vi "Read Multiple.vi"(8 "error in (no error)":errorcluster, 10 "Names":string[](array[string]), 11 "TwinCAT ADS in":refnum<class "TwinCAT ADS.lvclass">) -> (0 "error out":errorcluster, 1 "Values":variant[](array[variant]), 3 "TwinCAT ADS out":refnum<class "TwinCAT ADS.lvclass">)   [LabVIEW 2018, in "TwinCAT ADS.lvclass"]
uses:
  TwinCAT ADS.lvclass
  TwinCAT.Ads
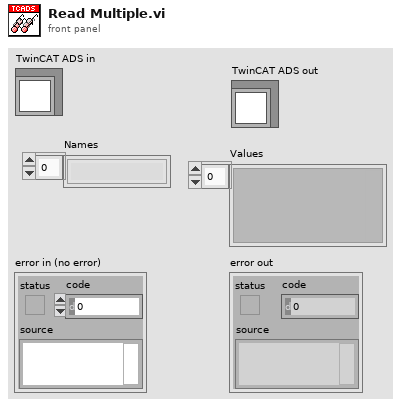
[diagram p1: front panel]
types:
  T1 = typedef "TwinCAT ADS.lvclass/Symbol Information.ctl" = cluster{"Name":string, "Short Name":string, "Size":i32, "Type Category":i32, "Type Name":string, "Type ID":i32, "Index Group":i64, "Index Offset":i64, "Child Count":i32, "Has Rpc Methods?":bool, "Comment":string}
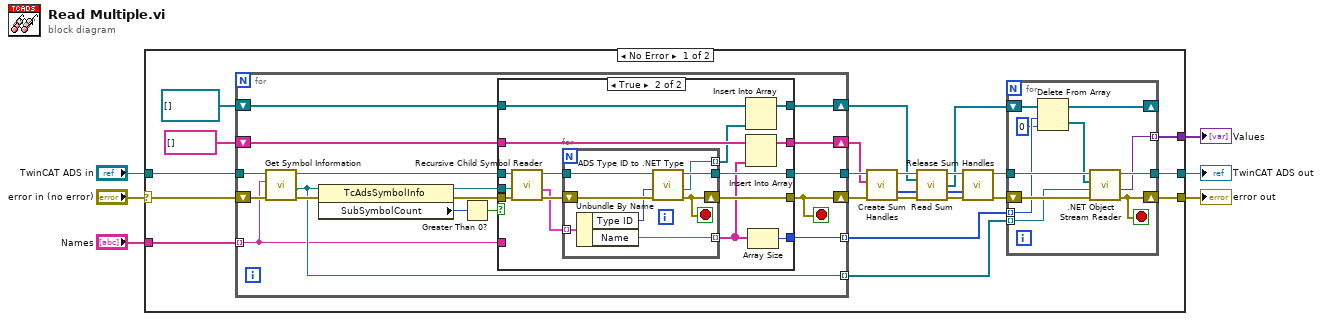
[diagram p0: block diagram]
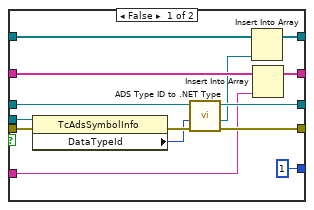
[diagram p2: hidden frame]
diagram:
  n1 = case shown="No Error" "error in (no error)" {
    selector: "error in (no error)" -> [w7 w96]
    tunnel: [w14 w96] -> w5
    tunnel: [w13 w95] -> w3
    tunnel: "TwinCAT ADS in" -> [w8 w95]
    tunnel: "Names" -> [w24 _]
    tunnel: [w12 _] -> w1
    frame No Error {
      n2 = for {
        tunnel: w24 -> [w41] mode=indexing
        shift-right: [w53] -> w26
        shift-left: string[] [] -> [w54]
        shift-right: [w52] -> w28
        shift-left: w7 -> [w46]
        tunnel: w8 -> [w45]
        tunnel: [w51] -> w27
        shift-right: [w48] -> w10
        shift-left: refnum<k24>[] [] (".NET Type Stream") -> [w50]
        tunnel: [w43] -> w11 mode=indexing
        tunnel: [w47] -> w15 mode=indexing
        stop <- w52 stop-if-true
        n3 = call-dynamic "Get Symbol Information.vi"("error in (no error)"=w46, "Name"=w41, "TwinCAT ADS in"=w45) -> ("error out"=w44:errorcluster, "Symbol Info"=w43:refnum<k24>, "TwinCAT ADS out"=w42:refnum<class "TwinCAT ADS.lvclass">)  [unwired: 6 in]
        n4 = property class="TcAdsSymbolInfo"(reference=w43, error in=w44) -> (reference out=w56:refnum<k24>, error out=w55:errorcluster, "SubSymbolCount"=w49:i32)
        n5 = Greater Than 0?(x=w49) -> (x > 0?=w57:bool)
        n6 = case shown="True" w57 {
          tunnel: w56 -> [w59 w84]
          tunnel: w55 -> [w69 w86]
          tunnel: [w63 w77] -> w52
          tunnel: [w70 w82] -> w53
          tunnel: w42 -> [w68 w85]
          tunnel: [w62 w76] -> w51
          tunnel: w54 -> [w71 w83]
          tunnel: w41 -> [w60 _]
          tunnel: w50 -> [w65 w81]
          tunnel: [w64 w74] -> w48
          tunnel: [1 w72] -> w47
          frame False {
            n7 = property class="TcAdsSymbolInfo"(reference=w59, error in=w69) -> (error out=w67:errorcluster, "DataTypeId"=w66:i32)  [unwired: 1 out]
            n8 = call "ADS Type ID to .NET Type.vi"("error in (no error)"=w67, "Type ID"=w66, "TwinCAT ADS in"=w68) -> ("error out"=w63:errorcluster, ".NET Type"=w61:refnum<k24>, "TwinCAT ADS out"=w62:refnum<class "TwinCAT ADS.lvclass">)  [unwired: 6 in]
            n9 = Insert Into Array(array=w65, new element=w61) -> (w64:refnum<k24>[])  [unwired: 1 in]
            n10 = Insert Into Array(array=w71, new element=w60) -> (w70:string[])  [unwired: 1 in]
          }
          frame True {
            n11 = call "Recursive Child Symbol Reader.vi"("error in (no error)"=w86, ".NET TcAdsSymbolInfo"=w84, "TwinCAT ADS in"=w85) -> ("error out"=w80:errorcluster, "Symbols Information"=w78:T1[], "TwinCAT ADS out"=w79:refnum<class "TwinCAT ADS.lvclass">)  [unwired: 6 in]
            n12 = for {
              tunnel: w78 -> [w94] mode=indexing
              tunnel: [w93] -> w73 mode=indexing
              shift-right: [w88] -> w77
              shift-left: w80 -> [w92]
              tunnel: w79 -> [w90]
              tunnel: [w89] -> w76
              tunnel: [w87] -> w75 mode=indexing
              stop <- w88 stop-if-true
              n13 = Unbundle By Name(w94) -> ("Type ID"=w91:i32, "Name"=w93:string)
              n14 = call "ADS Type ID to .NET Type.vi"("error in (no error)"=w92, "Type ID"=w91, "TwinCAT ADS in"=w90) -> ("error out"=w88:errorcluster, ".NET Type"=w87:refnum<k24>, "TwinCAT ADS out"=w89:refnum<class "TwinCAT ADS.lvclass">)  [unwired: 6 in]
            }
            n15 = Insert Into Array(array=w81, new element=w75) -> (w74:refnum<k24>[])  [unwired: 1 in]
            n16 = Insert Into Array(array=w83, new element=w73) -> (w82:string[])  [unwired: 1 in]
            n17 = Array Size(array=w73) -> (size(s)=w72:i32)
          }
        }
      }
      n18 = call-dynamic "Create Sum Handles.vi"("error in (no error)"=w28, "Names"=w26, "TwinCAT ADS in"=w27) -> ("error out"=w23:errorcluster, "Handles"=w22:u32[], "TwinCAT ADS out"=w21:refnum<class "TwinCAT ADS.lvclass">)  [unwired: 6 in]
      n19 = call-dynamic "Read Sum.vi"("TwinCAT ADS in"=w21, ".NET Type Stream"=w10, "Handles"=w22, "error in (no error)"=w23) -> ("TwinCAT ADS out"=w18:refnum<class "TwinCAT ADS.lvclass">, ".NET Object Stream"=w9:refnum<k24>[], "Handles"=w19:u32[], "error out"=w20:errorcluster)  [unwired: 8 in]
      n20 = call-dynamic "Release Sum Handles.vi"("error in (no error)"=w20, "Handles"=w19, "TwinCAT ADS in"=w18) -> ("error out"=w17:errorcluster, "TwinCAT ADS out"=w16:refnum<class "TwinCAT ADS.lvclass">)  [unwired: 7 in]
      n21 = for {
        tunnel: w11 -> [w38] mode=indexing
        tunnel: w16 -> [w40]
        tunnel: w15 -> [w32] mode=indexing
        shift-right: [w33] -> _
        shift-left: w9 -> [w34]
        shift-right: [w37] -> w14
        shift-left: w17 -> [w39]
        tunnel: [w36] -> w13
        tunnel: [w35] -> w12 mode=indexing
        stop <- w37 stop-if-true
        n22 = Delete From Array(array=w34, length=w32, index=0) -> (deleted portion=w30:refnum<k24>[], array with subset deleted=w33:refnum<k24>[])
        n23 = call-dynamic ".NET Object Stream Reader.vi"("error in (no error)"=w39, ".NET TcAdsSymbolInfo"=w38, ".NET Object Stream"=w30, "TwinCAT ADS in"=w40) -> ("error out"=w37:errorcluster, "G Object"=w35:variant, "TwinCAT ADS out"=w36:refnum<class "TwinCAT ADS.lvclass">)  [unwired: 5 in]
      }
    }
    frame Error {
    }
  }
  "error out" <- w5
  "TwinCAT ADS out" <- w3
  "Values" <- w1
